vi "To Serial Form.vi"(6 "Serial Version":T1, 10 "Serializer in":refnum<class "Serializer.lvclass">, 11 "PAS Cell Data in":refnum<class "PAS Cell Data.lvclass">) -> (0 "error out":errorcluster, 2 "Serializer out":refnum<class "Serializer.lvclass">, 3 "PAS Cell Data out":refnum<class "PAS Cell Data.lvclass">)   [LabVIEW 2014, in "PAS Cell Data.lvclass"]
uses:
  PAS Cell Data.lvclass
  <vilib>/NI/AQ Character Lineator/Serializer/Serializer.lvclass
  <vilib>/NI/AQ Character Lineator/Serialization Common/Serial Version.ctl
  PAS Cell Data.lvclass/PAS Cell Data.ctl
  <vilib>/NI/AQ Character Lineator/Serializable/Insert Double Array.vi
  <vilib>/NI/AQ Character Lineator/Serializable/Insert Double.vi
  <vilib>/NI/AQ Character Lineator/Serializer/Insert Double Array.vi
  <vilib>/NI/AQ Character Lineator/Serializer/Insert Double.vi
  <vilib>/NI/AQ Character Lineator/Serializer/Read Include Default Values.vi
  <vilib>/Analysis/Matrix/Numeric/Conversions/Matrix To Array - RM.vi
  Data/Data.lvclass
  <vilib>/NI/AQ Character Lineator/Serializable/Serializable.lvclass
  <vilib>/NI/AQ Character Lineator/Serializable Analog Waveform/Serializable Analog Waveform.lvclass
  <vilib>/Analysis/Matrix/NI_Matrix.lvlib
  <vilib>/NI/AQ Character Lineator/Serialization Common/Serialization Common.lvlib
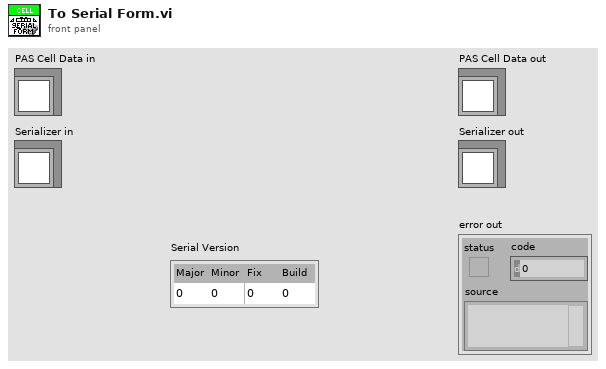
[diagram p1: front panel]
types:
  T1 = typedef "Serialization Common.lvlib/Serial Version.ctl" = cluster{"Major":u16, "Minor":u16, "Fix":u16, "Build":u16}
  T2 = typedef "NI_Matrix.lvlib/RealMatrix.ctl" = dbl[][]
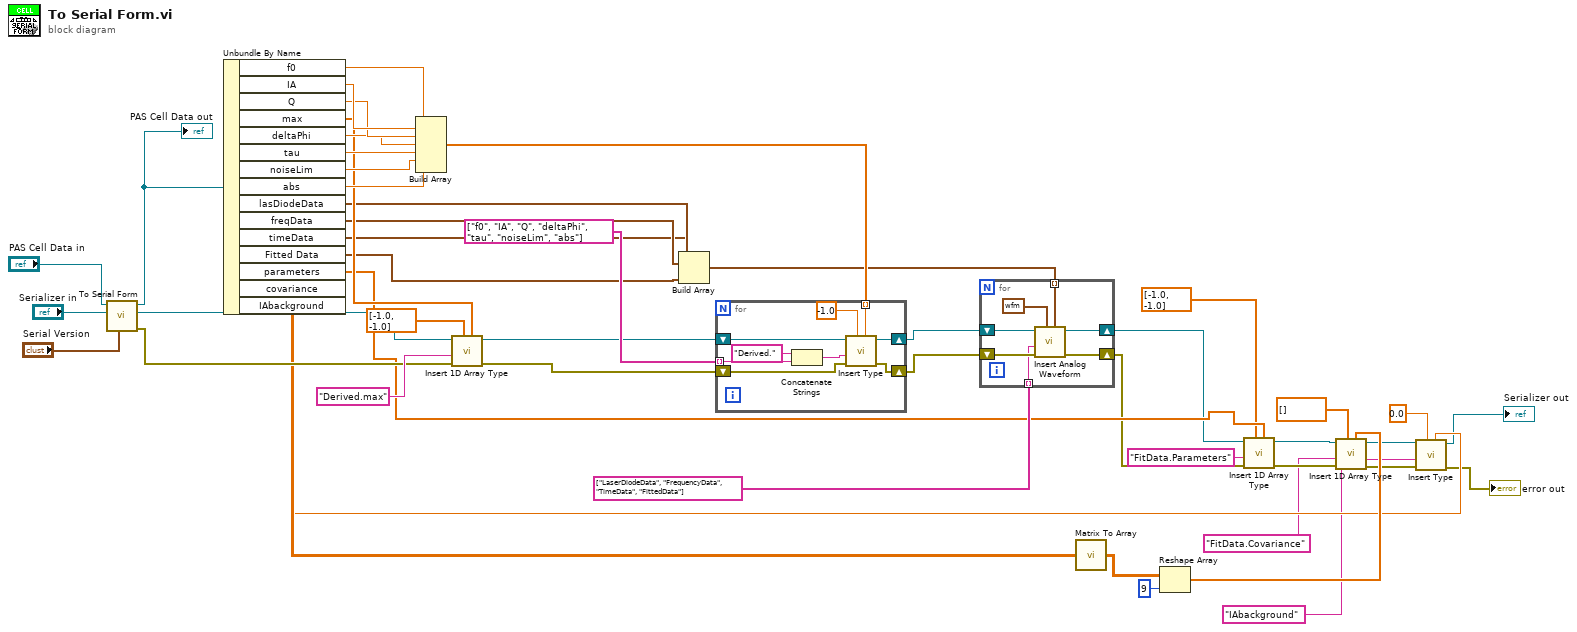
[diagram p0: block diagram]
diagram:
  n1 = call-parent "To Serial Form.vi"("Serial Version"="Serial Version", "Serializer in"="Serializer in", "Data in"="PAS Cell Data in") -> ("error out"=w33:errorcluster, "Serializer out"=w35:refnum<class "Serializer.lvclass">, "Data out"=w45:refnum<class "PAS Cell Data.lvclass">)  [unwired: 6 in]
  "PAS Cell Data out" <- w45
  n2 = Unbundle By Name(w45) -> ("f0"=w44:sgl, "IA"=w43:sgl, "Q"=w42:sgl, "max"=w37:dbl[], "deltaPhi"=w41:dbl, "tau"=w40:dbl, "noiseLim"=w39:dbl, "abs"=w38:dbl, "lasDiodeData"=w27:waveform(i16), "freqData"=w26:waveform(sgl), "timeData"=w25:waveform(i16), "Fitted Data"=w24:waveform(sgl), "parameters"=w20:dbl[], "covariance"=w13:T2, "IAbackground"=w6:dbl)
  n3 = Build Array(w44, w43, w42, w41, w40, w39, w38) -> (w32:dbl[])
  n4 = call-poly <vilib>:"Insert 1D Array Type.vi"("Doubles"=w37, "Default Value"=dbl[] [-1.0, -1.0], "error in (no error)"=w33, "Name"="Derived.max", "Serializer in"=w35) -> ("error out"=w29:errorcluster, "Serializer out"=w30:refnum<class "Serializer.lvclass">)  [unwired: 5 in]
  n5 = Build Array(w27, w26, w25, w24) -> (w23:waveform(sgl)[])
  n6 = for {
    tunnel: w32 -> [w57] mode=indexing
    tunnel: string[] ["f0", "IA", "Q", "deltaPhi", "tau", "noiseLim", "abs"] -> [w56] mode=indexing
    shift-right: [w53] -> w28
    shift-left: w30 -> [w54]
    shift-right: [w50] -> w22
    shift-left: w29 -> [w51]
    n7 = Concatenate Strings("Derived." ("string"), w56) -> (w52:string)
    n8 = call-poly <vilib>:"Insert Type.vi"("Double"=w57, "Default Value"=-1.0, "error in (no error)"=w51, "Name"=w52, "Serializer in"=w54) -> ("error out"=w50:errorcluster, "Serializer out"=w53:refnum<class "Serializer.lvclass">)  [unwired: 5 in]
  }
  n9 = for {
    shift-right: [w63] -> w19
    shift-left: w28 -> [w64]
    tunnel: w23 -> [w62] mode=indexing
    shift-right: [w59] -> w18
    shift-left: w22 -> [w60]
    tunnel: string[] ["LaserDiodeData", "FrequencyData", "TimeData", "FittedData"] -> [w58] mode=indexing
    n10 = call <vilib>:"Insert Analog Waveform.vi"("Analog Waveform"=w62, "Default Value"=waveform(dbl) {"t0"=timestamp(0 s since 1904-01-01), "dt"=1.0, "Y"=[]}, "error in (no error)"=w60, "Name"=w58, "Serializer in"=w64) -> ("error out"=w59:errorcluster, "Serializer out"=w63:refnum<class "Serializer.lvclass">)  [unwired: 5 in]
  }
  n11 = call-poly <vilib>:"Matrix To Array.vi"("Real Matrix"=w13) -> ("Real 2D Array"=w12:dbl[][])
  n12 = Reshape Array(w12, 9 ("dimension size")) -> (w11:dbl[])
  n13 = call-poly <vilib>:"Insert 1D Array Type.vi"("Doubles"=w20, "Default Value"=dbl[] [-1.0, -1.0], "error in (no error)"=w18, "Name"="FitData.Parameters", "Serializer in"=w19) -> ("error out"=w14:errorcluster, "Serializer out"=w15:refnum<class "Serializer.lvclass">)  [unwired: 5 in]
  n14 = call-poly <vilib>:"Insert 1D Array Type.vi"("Doubles"=w11, "Default Value"=dbl[] [], "error in (no error)"=w14, "Name"="FitData.Covariance", "Serializer in"=w15) -> ("error out"=w7:errorcluster, "Serializer out"=w8:refnum<class "Serializer.lvclass">)  [unwired: 5 in]
  n15 = call-poly <vilib>:"Insert Type.vi"("Double"=w6, "Default Value"=0.0, "error in (no error)"=w7, "Name"="IAbackground", "Serializer in"=w8) -> ("error out"=→"error out":errorcluster, "Serializer out"=→"Serializer out":refnum<class "Serializer.lvclass">)  [unwired: 5 in]
